vi "Start Pulse Measurements.vi"(8 "error in (no error)":errorcluster, 9 "Repeat times":i32=1, 10 "Objects":string[](array[string]), 11 "Monitor-Pulse in":refnum<class "Monitor-Pulse.lvclass">) -> (0 "error out":errorcluster, 3 "Monitor-Pulse out":refnum<class "Monitor-Pulse.lvclass">)   [LabVIEW 2015, in "Monitor-Pulse.lvclass"]
uses:
  Monitor-Pulse.lvclass
  Measure Controller Messages/Start Measurements Msg/Start Measurements Msg.lvclass/Start Measurements Msg.ctl
  <vilib>/ActorFramework/Message Enqueuer/Message Enqueuer.lvclass/Message Enqueuer.ctl
  <vilib>/ActorFramework/Message Enqueuer/Enqueue.vi
  <vilib>/ActorFramework/Message Priority Queue/Priority Enqueue.vi
  Measure Controller Messages/Start Measurements Msg/Start Measurements Msg.lvclass
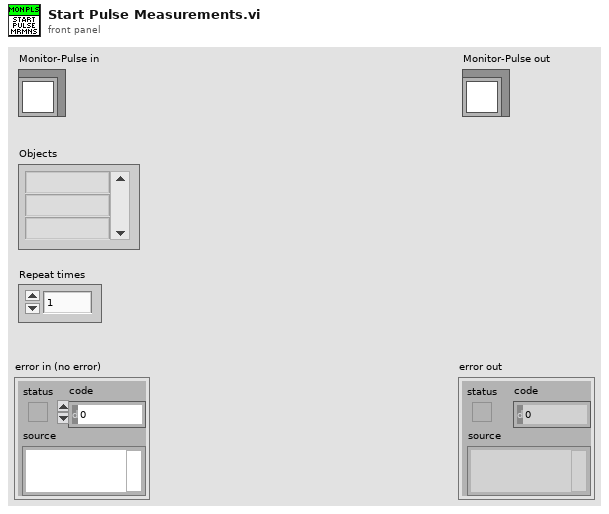
[diagram p1: front panel]
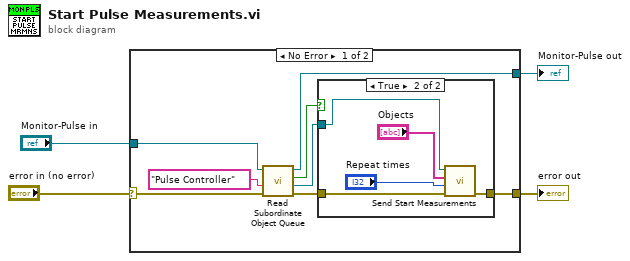
[diagram p0: block diagram]
diagram:
  n1 = case shown="No Error" "error in (no error)" {
    selector: "error in (no error)" -> [w9 w20]
    tunnel: [w5 w20] -> w3
    tunnel: [w11 w19] -> w1
    tunnel: "Monitor-Pulse in" -> [w12 w19]
    frame No Error {
      n2 = call-dynamic "Read Subordinate Object Queue.vi"("error in (no error)"=w9, "Name"="Pulse Controller", "Measure Object in"=w12) -> ("error out"=w6:errorcluster, "Object Enqueuer"=w8:refnum<class "Message Enqueuer.lvclass">, "Found?"=w7:bool, "Measure Object out"=w11:refnum<class "Monitor-Pulse.lvclass">)  [unwired: 5 in]
      n3 = case shown="True" w7 {
        tunnel: w8 -> [_ w18]
        tunnel: w6 -> [w13 w17]
        tunnel: [w13 w14] -> w5
        frame False {
        }
        frame True {
          n4 = call "Send Start Measurements.vi"("error in (no error)"=w17, "Repeat times"="Repeat times", "Objects"="Objects", "Message Enqueuer"=w18) -> ("error out"=w14:errorcluster)  [unwired: 6 in, 1 out]
        }
      }
    }
    frame Error {
    }
  }
  "error out" <- w3
  "Monitor-Pulse out" <- w1
